vi "SYST.vi"(8 "error in (no error)":errorcluster, 11 "FTP in":refnum<class "FTP.lvclass">) -> (0 "error out":errorcluster, 3 "FTP out":refnum<class "FTP.lvclass">)   [LabVIEW 2017, in "FTP.lvlib" / "FTP.lvclass"]
uses:
  FTP.lvclass
  FTP.lvclass/FTP.ctl
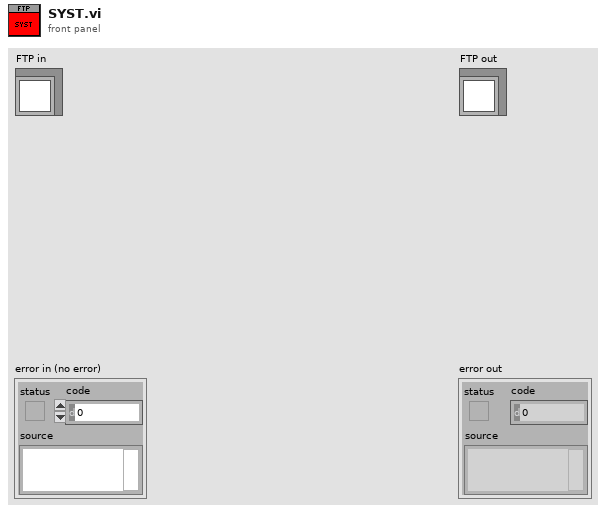
[diagram p1: front panel]
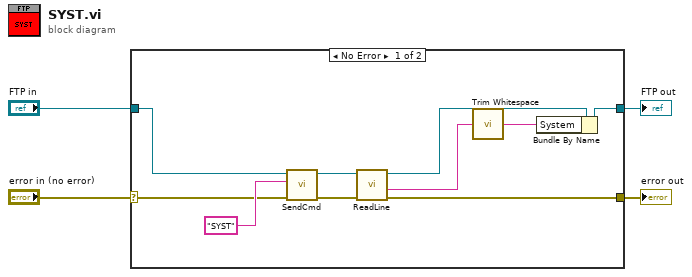
[diagram p0: block diagram]
diagram:
  n1 = case shown="No Error" "error in (no error)" {
    selector: "error in (no error)" -> [w10 w16]
    tunnel: [w9 w16] -> w3
    tunnel: [w7 w15] -> w1
    tunnel: "FTP in" -> [w11 w15]
    frame No Error {
      n2 = call "SendCmd.vi"("error in (no error)"=w10, "cmd"="SYST", "FTP in"=w11) -> ("error out"=w14:errorcluster, "FTP out"=w13:refnum<class "FTP.lvclass">)  [unwired: 7 in]
      n3 = call "ReadLine.vi"("error in (no error)"=w14, "FTP in"=w13) -> ("error out"=w9:errorcluster, "Line"=w6:string, "FTP out"=w8:refnum<class "FTP.lvclass">)  [unwired: 5 in, 2 out]
      n4 = call <vilib>:"Trim Whitespace.vi"("string"=w6) -> ("trimmed string"=w5:string)  [unwired: 1 in]
      n5 = Bundle By Name(cluster=w8, "System"=w5) -> (w7:refnum<class "FTP.lvclass">)
    }
    frame Error {
    }
  }
  "error out" <- w3
  "FTP out" <- w1
